vi "MusicEmotionControl.vi"(6 "Roll off":dbl, 7 "Centroid":dbl, 9 "Zero Crossing":dbl, 10 "RMS":dbl, 11 "BPM":dbl) -> (1 "XY Graph":cluster{"Y":dbl[], "Y":dbl[]}[](graph) caption="XY 그래프", 2 "흥분도":dbl format="%.2g", 3 "행복도":dbl format="%.2g")   [LabVIEW 2020]
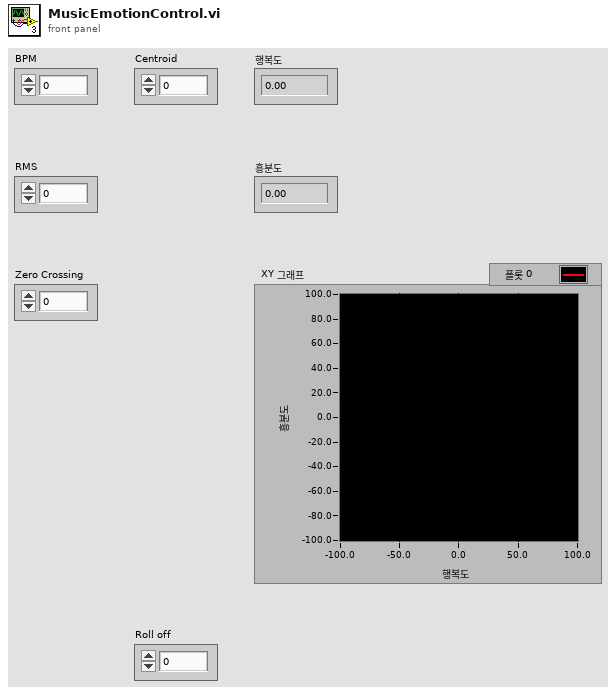
[diagram p1: front panel]
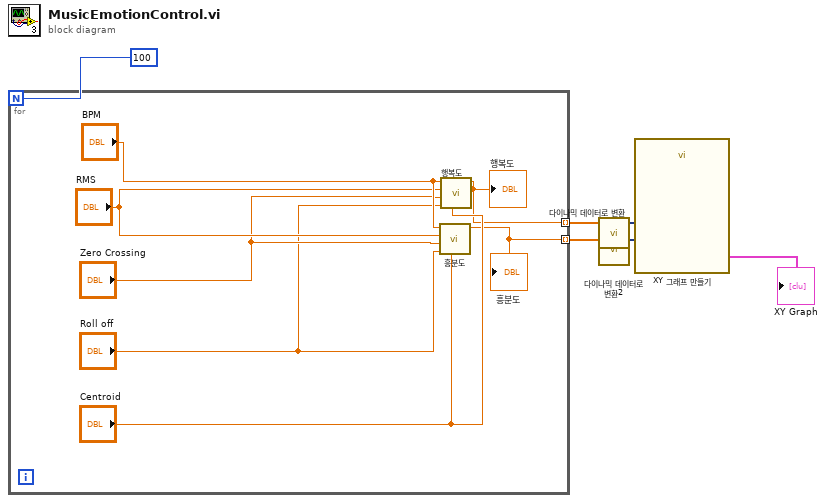
[diagram p0: block diagram]
diagram:
  n1 = for {
    N: 100 -> [_]
    tunnel: [w8] -> w3 mode=indexing
    tunnel: [w7] -> w5 mode=indexing
    n2 = call "흥분도.vi"("밝기"="Centroid", "진폭변화"="Roll off", "잡음"="Zero Crossing", "역동성"="RMS", "템포"="BPM") -> ("흥분도"=w7:dbl)  [unwired: 6 in]
    "흥분도" <- w7
    n3 = call "행복도.vi"("밝기"="Centroid", "진폭변화"="Roll off", "잡음"="Zero Crossing", "역동성"="RMS", "템포"="BPM") -> ("행복도"=w8:dbl)  [unwired: 6 in]
    "행복도" <- w8
  }
  n4 = call "다이나믹 데이터로 변환"("Array"=w3) -> ("Dynamic Data Type"=w4:dynamicdata)  [unwired: 3 in]
  n5 = call "다이나믹 데이터로 변환2"("Array"=w5) -> ("Dynamic Data Type"=w6:dynamicdata)  [unwired: 3 in]
  n6 = call "XY 그래프 만들기"("Y Input"=w6, "X Input"=w4) -> ("XY Graph"=→"XY Graph":cluster{"X":dbl[], "Y":dbl[]}[])  [unwired: 8 in, 1 out]
